vi "solar_excel Cell Truncate.vi"(11 "Cells in":string[][](array[string])) -> (3 "Truncated Cells out":string[][](array[string]))   [LabVIEW 2018]
doc: "This truncates any empty strings and the end of the 2D array."
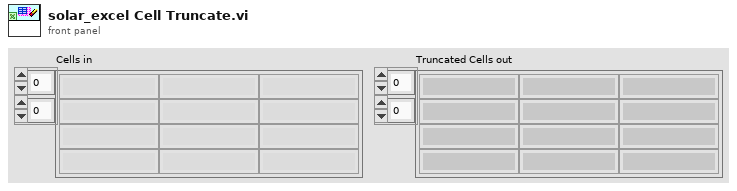
[diagram p1: front panel]
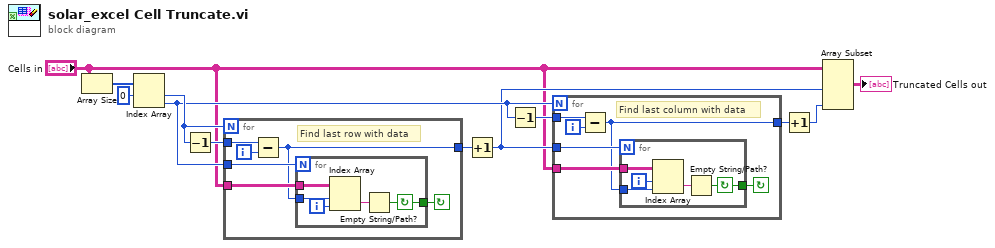
[diagram p0: block diagram]
diagram:
  n1 = Array Size(array="Cells in") -> (size(s)=w12:i32[])
  n2 = Index Array(array=w12, index #1=0 ("index")) -> (element #1=w10:i32, element #2=w7:i32)  [unwired: 1 in]
  n3 = Decrement(x=w10) -> (x-1=w9:i32)
  n4 = for {
    N: w10 -> [_]
    tunnel: "Cells in" -> [w17]
    tunnel: w9 -> [w16]
    tunnel: w7 -> [w18]
    tunnel: [w13] -> w8
    i -> [w14]
    stop <- w15 continue-if-true
    # "Find last row with data"
    n5 = Subtract(x=w16, y=w14) -> (x-y=w13:i32)
    n6 = for {
      N: w18 -> [_]
      tunnel: w17 -> [w23]
      tunnel: w13 -> [w22]
      tunnel: [w19] -> w15
      i -> [w20]
      stop <- w19 continue-if-true
      n7 = Index Array(array=w23, index (row)=w22, index (col)=w20) -> (element=w21:string)
      n8 = Empty String/Path?(string/path=w21) -> (empty?=w19:bool)
    }
  }
  n9 = Increment(x=w8) -> (x+1=w4:i32)
  n10 = Decrement(x=w7) -> (x-1=w6:i32)
  n11 = for {
    N: w7 -> [_]
    tunnel: "Cells in" -> [w28]
    tunnel: w6 -> [w27]
    tunnel: w4 -> [w29]
    tunnel: [w24] -> w5
    i -> [w25]
    stop <- w26 continue-if-true
    # "Find last column with data"
    n12 = Subtract(x=w27, y=w25) -> (x-y=w24:i32)
    n13 = for {
      N: w29 -> [_]
      tunnel: w28 -> [w34]
      tunnel: w24 -> [w30]
      tunnel: [w32] -> w26
      i -> [w31]
      stop <- w32 continue-if-true
      n14 = Index Array(array=w34, index (row)=w31, index (col)=w30) -> (element=w33:string)
      n15 = Empty String/Path?(string/path=w33) -> (empty?=w32:bool)
    }
  }
  n16 = Increment(x=w5) -> (x+1=w3:i32)
  n17 = Array Subset(array="Cells in", length (row)=w4, length (col)=w3) -> (→"Truncated Cells out":string[][])  [unwired: 2 in]
